vi "First SubVI.vi"(11 "logger in":refnum<class "Logger.lvclass">) -> (3 "logger out":refnum<class "Logger.lvclass">)   [LabVIEW 2018, in "Scope Tester Library.lvlib" / "Scope Tester Class.lvclass"]
uses:
  Scope Tester Class.lvclass
  Logger/Logger.lvclass
  Log Levels.ctl
  Logging.lvlib
  Scope Tester Library.lvlib
panel:
  # "Connector Pane"
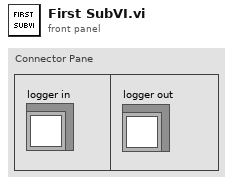
[diagram p1: front panel]
types:
  T1 = typedef "Logging.lvlib/Log Levels.ctl" = enum16{"Trace", "Debug", "Info", "Warning", "Error", "Critical"}
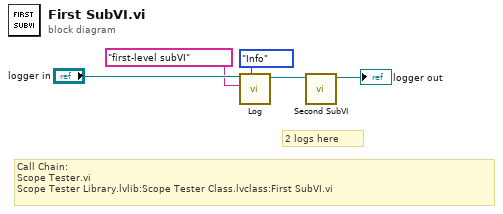
[diagram p0: block diagram]
diagram:
  # "2 logs here"
  # "Call Chain: \nScope Tester.vi\nScope Tester Library.lvlib:Scope Tester Class.lvclass:First SubVI.vi"
  n1 = call "Log.vi"("log level"=Log_Levels."Info" ("level"), "message"="first-level subVI", "logger in"="logger in") -> ("logger out"=w5:refnum<class "Logger.lvclass">)  [unwired: 8 in]
  n2 = call "Second SubVI.vi"("logger in"=w5) -> ("logger out"=→"logger out":refnum<class "Logger.lvclass">)  [unwired: 10 in]
